vi "FUG-HCN.ProcEvents.vi"(0 "i ref in":refnum<vi>, 5 "error in":errorcluster) -> (14 "i ref out":refnum<vi>, 19 "error out":errorcluster)   [LabVIEW 2014, in "FUG-HCN.lvlib"]
doc: "This method is used to define the events the object will listen to. Add your own events here."
uses:
  FUG-HCN.lvlib
  CSCore/BaseProcess/BaseProcess.event definition.ctl
  CSCore/CAEObj/CAEObj.event definition.ctl
  CSCore/BaseProcess/BaseProcess.descriptor string definition.ctl
  CSCore/BaseProcess/BaseProcess.lvlib
  CSCore/CAEObj/CAEObj.lvlib
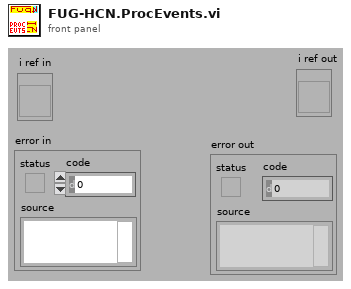
[diagram p1: front panel]
types:
  T1 = typedef "BaseProcess.lvlib/BaseProcess.event definition.ctl" = cluster{"CAEEvtDef":T2, "Data Descriptor":T3}
  T2 = typedef "CAEObj.lvlib/CAEObj.event definition.ctl" = cluster{"URL":string, "enable":bool, "ignoreResID":bool}
  T3 = typedef "BaseProcess.lvlib/BaseProcess.descriptor string definition.ctl" = string
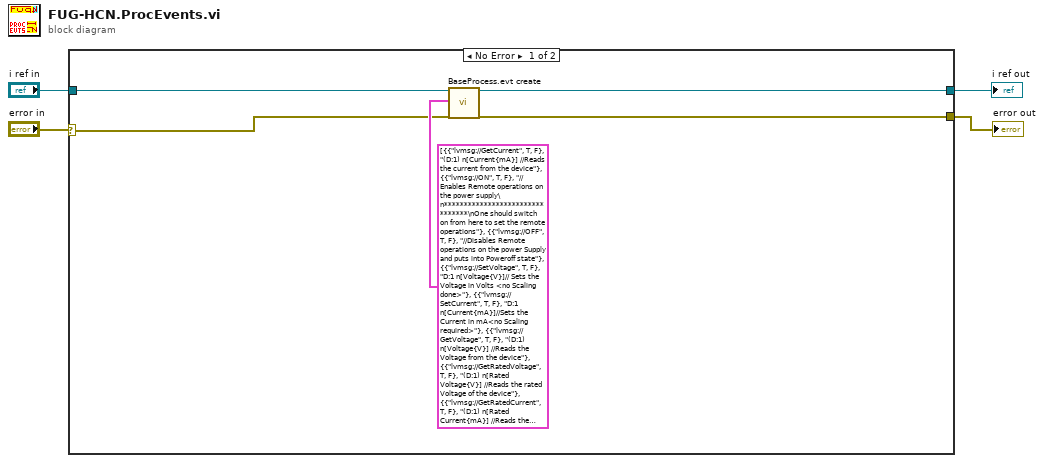
[diagram p0: block diagram]
diagram:
  n1 = case shown="No Error" "error in" {
    selector: "error in" -> [w5 w11]
    tunnel: "i ref in" -> [w9 w10]
    tunnel: [w8 w11] -> w3
    tunnel: [w7 w10] -> w2
    frame No Error {
      n2 = call "BaseProcess.evt create.vi"("i ref in"=w9, "newEvents"=T1[] [{"CAEEvtDef"={"URL"="lvmsg://GetCurrent", "enable"=TRUE, "ignoreResID"=FALSE}, "Data Descriptor"="(D:1) n[Current{mA}] //Reads the current from the device"}, {"CAEEvtDef"={"URL"="lvmsg://ON", "enable"=TRUE, "ignoreResID"=FALSE}, "Data Descriptor"="//Enables Remote operations on the power supply\n********************************\nOne should switch on from here to set the remote operations"}, {"CAEEvtDef"={"URL"="lvmsg://OFF", "enable"=TRUE, "ignoreResID"=FALSE}, "Data Descriptor"="//Disables Remote operations on the power Supply and puts into Poweroff state"}, {"CAEEvtDef"={"URL"="lvmsg://SetVoltage", "enable"=TRUE, "ignoreResID"=FALSE}, "Data Descriptor"="D:1 n[Voltage{V}]// Sets the Voltage in Volts <no Scaling done>"}, {"CAEEvtDef"={"URL"="lvmsg://SetCurrent", "enable"=TRUE, "ignoreResID"=FALSE}, "Data Descriptor"="D:1 n[Current{mA}]//Sets the Current in mA<no Scaling required>"}, {"CAEEvtDef"={"URL"="lvmsg://GetVoltage", "enable"=TRUE, "ignoreResID"=FALSE}, "Data Descriptor"="(D:1) n[Voltage{V}] //Reads the Voltage from the device"}, {"CAEEvtDef"={"URL"="lvmsg://GetRatedVoltage", "enable"=TRUE, "ignoreResID"=FALSE}, "Data Descriptor"="(D:1) n[Rated Voltage{V}] //Reads the rated Voltage of the device"}, {"CAEEvtDef"={"URL"="lvmsg://GetRatedCurrent", "enable"=TRUE, "ignoreResID"=FALSE}, "Data Descriptor"="(D:1) n[Rated Current{mA}] //Reads the rated current of the device"}, {"CAEEvtDef"={"URL"="lvmsg://Remote", "enable"=TRUE, "ignoreResID"=FALSE}, "Data Descriptor"="S:1 n[Remote {On,Off}] //Enables remote operation"}] ("new events"), "error in (no error)"=w5) -> ("i ref out"=w7:refnum<vi>, "error out"=w8:errorcluster)  [unwired: 13 in, 2 out]
    }
    frame Error {
    }
  }
  "i ref out" <- w2
  "error out" <- w3
